vi "state machine.vi"() -> ()   [LabVIEW 2012]
panel:
  out "case status":T1(ring)
  in  "stop":bool
  in  "start":bool
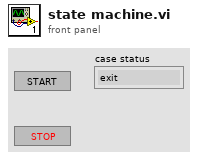
[diagram p1: front panel]
types:
  T1 = enum16{"exit", "1", "2", "3", "4", "5", "6", "7", "8", "9", "10", "initialize", "start"}
  T2 = enum16{"exit", "1", "2", "3", "4", "5", "6", "7", "8", "9", "10", "initialize", "start"}[]
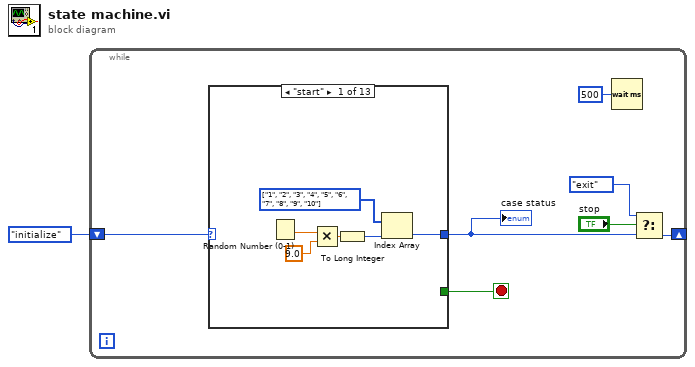
[diagram p0: block diagram]
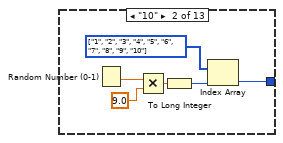
[diagram p2: hidden frame]
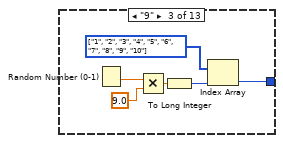
[diagram p3: hidden frame]
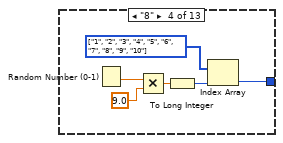
[diagram p4: hidden frame]
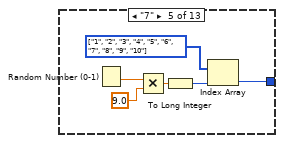
[diagram p5: hidden frame]
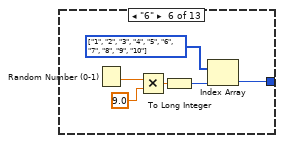
[diagram p6: hidden frame]
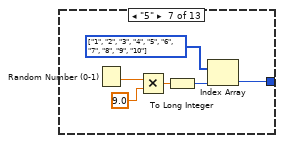
[diagram p7: hidden frame]
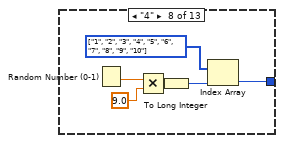
[diagram p8: hidden frame]
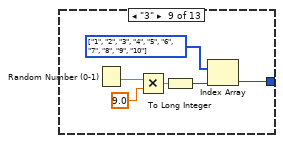
[diagram p9: hidden frame]
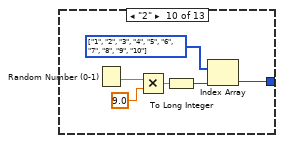
[diagram p10: hidden frame]
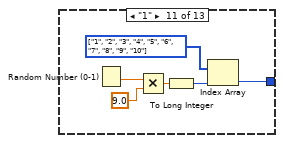
[diagram p11: hidden frame]
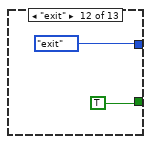
[diagram p12: hidden frame]
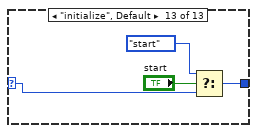
[diagram p13: hidden frame]
diagram:
  n1 = while {
    shift-right: [w5] -> _
    shift-left: T1."initialize" -> [w6]
    stop <- w3 stop-if-true
    n2 = case shown="\"start\"" w6 {
      selector: w6 -> [_ _ _ _ _ _ _ _ _ _ _ _ w79]
      tunnel: [w11 w17 w23 w29 w35 w41 w47 w53 w59 w65 w71 T1."exit" w80] -> w8
      tunnel: [_ _ _ _ _ _ _ _ _ _ _ TRUE _] -> w3
      frame "start" {
        w14 = T2 [enum."1", enum."2", enum."3", enum."4", enum."5", enum."6", enum."7", enum."8", enum."9", enum."10"] items=["exit", "1", "2", "3", "4", "5", "6", "7", "8", "9", "10", "initialize", "start"]
        n3 = Random Number (0-1)() -> (number: 0 to 1=w12:dbl)
        n4 = Multiply(x=w12, y=9.0) -> (x*y=w10:dbl)
        n5 = To Long Integer(number=w10) -> (32bit integer=w9:i32)
        n6 = Index Array(array=w14, index=w9) -> (element=w11:T1)
      }
      frame "10" {
        w20 = T2 [enum."1", enum."2", enum."3", enum."4", enum."5", enum."6", enum."7", enum."8", enum."9", enum."10"] items=["exit", "1", "2", "3", "4", "5", "6", "7", "8", "9", "10", "initialize", "start"]
        n7 = Random Number (0-1)() -> (number: 0 to 1=w18:dbl)
        n8 = Multiply(x=w18, y=9.0) -> (x*y=w16:dbl)
        n9 = To Long Integer(number=w16) -> (32bit integer=w15:i32)
        n10 = Index Array(array=w20, index=w15) -> (element=w17:T1)
      }
      frame "9" {
        w26 = T2 [enum."1", enum."2", enum."3", enum."4", enum."5", enum."6", enum."7", enum."8", enum."9", enum."10"] items=["exit", "1", "2", "3", "4", "5", "6", "7", "8", "9", "10", "initialize", "start"]
        n11 = Random Number (0-1)() -> (number: 0 to 1=w24:dbl)
        n12 = Multiply(x=w24, y=9.0) -> (x*y=w22:dbl)
        n13 = To Long Integer(number=w22) -> (32bit integer=w21:i32)
        n14 = Index Array(array=w26, index=w21) -> (element=w23:T1)
      }
      frame "8" {
        w32 = T2 [enum."1", enum."2", enum."3", enum."4", enum."5", enum."6", enum."7", enum."8", enum."9", enum."10"] items=["exit", "1", "2", "3", "4", "5", "6", "7", "8", "9", "10", "initialize", "start"]
        n15 = Random Number (0-1)() -> (number: 0 to 1=w30:dbl)
        n16 = Multiply(x=w30, y=9.0) -> (x*y=w28:dbl)
        n17 = To Long Integer(number=w28) -> (32bit integer=w27:i32)
        n18 = Index Array(array=w32, index=w27) -> (element=w29:T1)
      }
      frame "7" {
        w38 = T2 [enum."1", enum."2", enum."3", enum."4", enum."5", enum."6", enum."7", enum."8", enum."9", enum."10"] items=["exit", "1", "2", "3", "4", "5", "6", "7", "8", "9", "10", "initialize", "start"]
        n19 = Random Number (0-1)() -> (number: 0 to 1=w36:dbl)
        n20 = Multiply(x=w36, y=9.0) -> (x*y=w34:dbl)
        n21 = To Long Integer(number=w34) -> (32bit integer=w33:i32)
        n22 = Index Array(array=w38, index=w33) -> (element=w35:T1)
      }
      frame "6" {
        w44 = T2 [enum."1", enum."2", enum."3", enum."4", enum."5", enum."6", enum."7", enum."8", enum."9", enum."10"] items=["exit", "1", "2", "3", "4", "5", "6", "7", "8", "9", "10", "initialize", "start"]
        n23 = Random Number (0-1)() -> (number: 0 to 1=w42:dbl)
        n24 = Multiply(x=w42, y=9.0) -> (x*y=w40:dbl)
        n25 = To Long Integer(number=w40) -> (32bit integer=w39:i32)
        n26 = Index Array(array=w44, index=w39) -> (element=w41:T1)
      }
      frame "5" {
        w50 = T2 [enum."1", enum."2", enum."3", enum."4", enum."5", enum."6", enum."7", enum."8", enum."9", enum."10"] items=["exit", "1", "2", "3", "4", "5", "6", "7", "8", "9", "10", "initialize", "start"]
        n27 = Random Number (0-1)() -> (number: 0 to 1=w48:dbl)
        n28 = Multiply(x=w48, y=9.0) -> (x*y=w46:dbl)
        n29 = To Long Integer(number=w46) -> (32bit integer=w45:i32)
        n30 = Index Array(array=w50, index=w45) -> (element=w47:T1)
      }
      frame "4" {
        w56 = T2 [enum."1", enum."2", enum."3", enum."4", enum."5", enum."6", enum."7", enum."8", enum."9", enum."10"] items=["exit", "1", "2", "3", "4", "5", "6", "7", "8", "9", "10", "initialize", "start"]
        n31 = Random Number (0-1)() -> (number: 0 to 1=w54:dbl)
        n32 = Multiply(x=w54, y=9.0) -> (x*y=w52:dbl)
        n33 = To Long Integer(number=w52) -> (32bit integer=w51:i32)
        n34 = Index Array(array=w56, index=w51) -> (element=w53:T1)
      }
      frame "3" {
        w62 = T2 [enum."1", enum."2", enum."3", enum."4", enum."5", enum."6", enum."7", enum."8", enum."9", enum."10"] items=["exit", "1", "2", "3", "4", "5", "6", "7", "8", "9", "10", "initialize", "start"]
        n35 = Random Number (0-1)() -> (number: 0 to 1=w60:dbl)
        n36 = Multiply(x=w60, y=9.0) -> (x*y=w58:dbl)
        n37 = To Long Integer(number=w58) -> (32bit integer=w57:i32)
        n38 = Index Array(array=w62, index=w57) -> (element=w59:T1)
      }
      frame "2" {
        w68 = T2 [enum."1", enum."2", enum."3", enum."4", enum."5", enum."6", enum."7", enum."8", enum."9", enum."10"] items=["exit", "1", "2", "3", "4", "5", "6", "7", "8", "9", "10", "initialize", "start"]
        n39 = Random Number (0-1)() -> (number: 0 to 1=w66:dbl)
        n40 = Multiply(x=w66, y=9.0) -> (x*y=w64:dbl)
        n41 = To Long Integer(number=w64) -> (32bit integer=w63:i32)
        n42 = Index Array(array=w68, index=w63) -> (element=w65:T1)
      }
      frame "1" {
        w74 = T2 [enum."1", enum."2", enum."3", enum."4", enum."5", enum."6", enum."7", enum."8", enum."9", enum."10"] items=["exit", "1", "2", "3", "4", "5", "6", "7", "8", "9", "10", "initialize", "start"]
        n43 = Random Number (0-1)() -> (number: 0 to 1=w72:dbl)
        n44 = Multiply(x=w72, y=9.0) -> (x*y=w70:dbl)
        n45 = To Long Integer(number=w70) -> (32bit integer=w69:i32)
        n46 = Index Array(array=w74, index=w69) -> (element=w71:T1)
      }
      frame "exit" {
      }
      frame "initialize", Default {
        n47 = Select(t=T1."start", s="start", f=w79) -> (s? t:f=w80:T1)
      }
    }
    "case status" <- w8
    n48 = Wait (ms)(milliseconds to wait=u32 500) -> ()  [unwired: 1 out]
    n49 = Select(t=T1."exit", s="stop", f=w8) -> (s? t:f=w5:T1)
  }
